vi "read data - HP4192A Impedance Analyzer.vi"(0 "file path (dialog if empty)":path) -> (1 "Hz":dbl[](array[numeric]) format="%.2f", 2 "R":dbl[](array[numeric]) format="%.2f", 3 "X":dbl[](array[numeric]) format="%.2f", 4 "Temp":dbl[](array[numeric]) format="%.2f")   [LabVIEW 2012]
uses:
  <vilib>/Utility/file.llb/Read From Spreadsheet File (DBL).vi
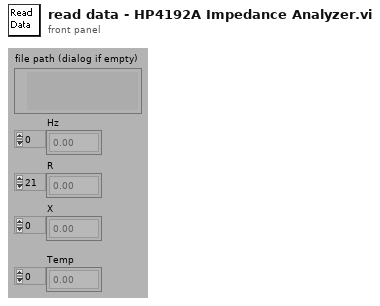
[diagram p1: front panel]
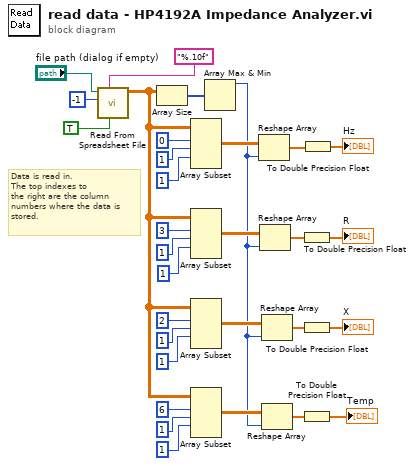
[diagram p0: block diagram]
diagram:
  # "Data is read in. \nThe top indexes to \nthe right are the column\nnumbers where the data is\nstored."
  n1 = call-poly <vilib>:"Read From Spreadsheet File.vi"("transpose (no:F)"=TRUE, "format (%.3f)"="%.10f", "number of rows (all:-1)"=-1, "file path (dialog if empty)"="file path (dialog if empty)") -> ("all rows"=w6:dbl[][])  [unwired: 3 in, 4 out]
  n2 = Array Size(array=w6) -> (size(s)=w27:i32[])
  n3 = Array Subset(array=w6, index (row)=0 ("index"), length (row)=1 ("length"), index (col)=1 ("length")) -> (w25:dbl[][])  [unwired: 1 in]
  n4 = Array Subset(array=w6, index (row)=3 ("index"), length (row)=1 ("length"), index (col)=1 ("length")) -> (w24:dbl[][])  [unwired: 1 in]
  n5 = Array Subset(array=w6, index (row)=2 ("index"), length (row)=1 ("length"), index (col)=1 ("length")) -> (w23:dbl[][])  [unwired: 1 in]
  n6 = Array Subset(array=w6, index (row)=6 ("index"), length (row)=1 ("length"), index (col)=1 ("length")) -> (w8:dbl[][])  [unwired: 1 in]
  n7 = Array Max & Min(array=w27) -> (max value=w7:i32)  [unwired: 3 out]
  n8 = Reshape Array(w25, w7) -> (w20:dbl[])
  n9 = Reshape Array(w24, w7) -> (w21:dbl[])
  n10 = Reshape Array(w23, w7) -> (w22:dbl[])
  n11 = Reshape Array(w8, w7) -> (w9:dbl[])
  n12 = To Double Precision Float(number=w21) -> (double precision float=→"R":dbl[])
  n13 = To Double Precision Float(number=w22) -> (double precision float=→"X":dbl[])
  n14 = To Double Precision Float(number=w9) -> (double precision float=→"Temp":dbl[])
  n15 = To Double Precision Float(number=w20) -> (double precision float=→"Hz":dbl[])
